vi "subcontrolmotor.vi"(0 "Boolesch":bool) -> ()   [LabVIEW 2011]
uses:
  <vilib>/DAQmx/write.llb/DAQmx Write (Digital Bool 1Line 1Point).vi
  <vilib>/DAQmx/create/channels.llb/DAQmx Create Channel (DO-Digital Output).vi
  <vilib>/DAQmx/miscellaneous.llb/DAQmx Fill In Error Info.vi
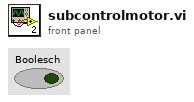
[diagram p1: front panel]
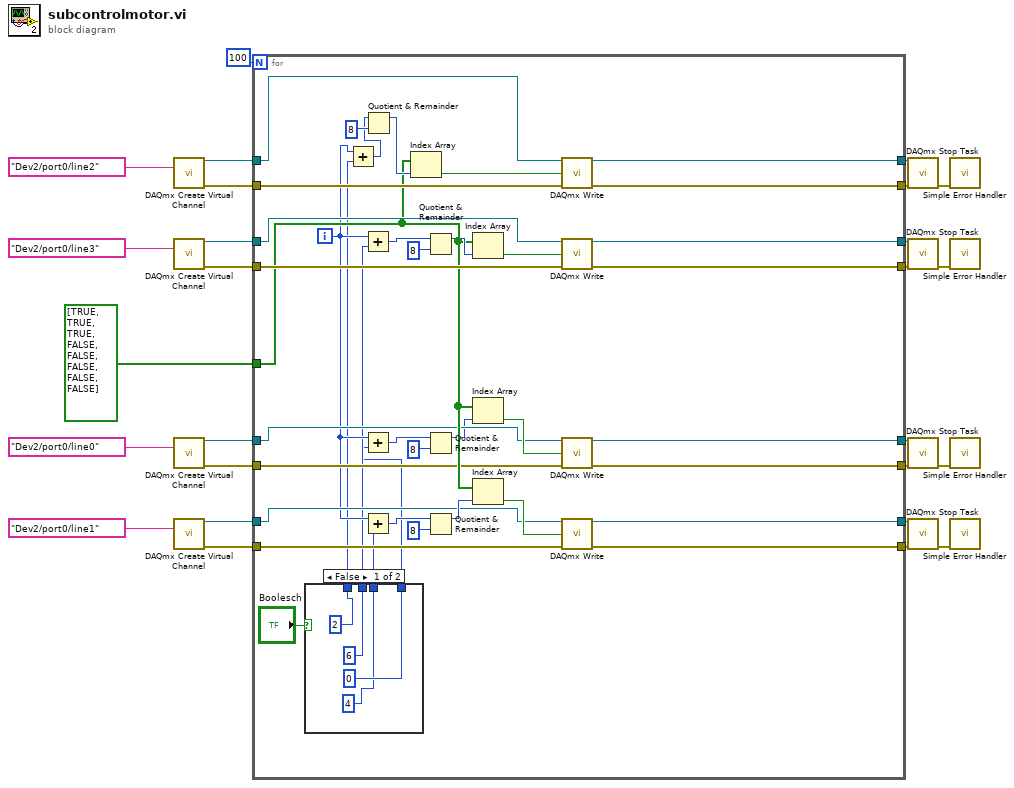
[diagram p0: block diagram]
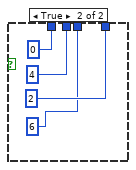
[diagram p2: hidden frame]
diagram:
  n1 = call-poly <vilib>:"DAQmx Create Virtual Channel.vi"("lines"=tag "Dev2/port0/line2") -> ("task out"=w26:refnum<k21>, "error out"=w25:errorcluster)  [unwired: 13 in]
  n2 = call-poly <vilib>:"DAQmx Create Virtual Channel.vi"("lines"=tag "Dev2/port0/line3") -> ("task out"=w20:refnum<k21>, "error out"=w19:errorcluster)  [unwired: 13 in]
  n3 = call-poly <vilib>:"DAQmx Create Virtual Channel.vi"("lines"=tag "Dev2/port0/line0") -> ("task out"=w11:refnum<k21>, "error out"=w10:errorcluster)  [unwired: 13 in]
  n4 = call-poly <vilib>:"DAQmx Create Virtual Channel.vi"("lines"=tag "Dev2/port0/line1") -> ("task out"=w3:refnum<k21>, "error out"=w2:errorcluster)  [unwired: 13 in]
  n5 = for {
    N: 100 -> [_]
    tunnel: w26 -> [w65]
    tunnel: w25 -> [w64]
    tunnel: [w63] -> w24
    tunnel: [w62] -> w22
    tunnel: bool[] [TRUE, TRUE, TRUE, FALSE, FALSE, FALSE, FALSE, FALSE] -> [w50]
    tunnel: w20 -> [w54]
    tunnel: w19 -> [w53]
    tunnel: [w52] -> w17
    tunnel: [w51] -> w16
    tunnel: w11 -> [w47]
    tunnel: w10 -> [w46]
    tunnel: [w45] -> w8
    tunnel: [w44] -> w7
    tunnel: [w43] -> w5
    tunnel: [w42] -> w4
    tunnel: w3 -> [w35]
    tunnel: w2 -> [w34]
    i -> [w33]
    n6 = case shown="False" "Boolesch" {
      tunnel: [2 ("y") 0 ("y")] -> w30
      tunnel: [6 ("y") 4 ("y")] -> w29
      tunnel: [0 ("y") 2 ("y")] -> w28
      tunnel: [4 ("y") 6 ("y")] -> w27
      frame False {
      }
      frame True {
      }
    }
    n7 = Add(x=w33, y=w30) -> (x+y=w32:i32)
    n8 = Add(x=w33, y=w29) -> (x+y=w56:i32)
    n9 = Add(x=w33, y=w28) -> (x+y=w40:i32)
    n10 = Add(x=w33, y=w27) -> (x+y=w41:i32)
    n11 = Quotient & Remainder(x=w32, y=8) -> (x-y*floor(x/y)=w60:i32)  [unwired: 1 out]
    n12 = Index Array(array=w50, index=w60) -> (element=w59:bool)
    n13 = Quotient & Remainder(x=w56, y=8) -> (x-y*floor(x/y)=w58:i32)  [unwired: 1 out]
    n14 = Quotient & Remainder(x=w40, y=8) -> (x-y*floor(x/y)=w38:i32)  [unwired: 1 out]
    n15 = Quotient & Remainder(x=w41, y=8) -> (x-y*floor(x/y)=w39:i32)  [unwired: 1 out]
    n16 = Index Array(array=w50, index=w58) -> (element=w55:bool)
    n17 = Index Array(array=w50, index=w38) -> (element=w48:bool)
    n18 = Index Array(array=w50, index=w39) -> (element=w49:bool)
    n19 = call-poly <vilib>:"DAQmx Write.vi"("task/channels in"=w65, "data"=w59, "error in"=w64) -> ("task out"=w62:refnum<k21>, "error out"=w63:errorcluster)  [unwired: 10 in, 1 out]
    n20 = call-poly <vilib>:"DAQmx Write.vi"("task/channels in"=w54, "data"=w55, "error in"=w53) -> ("task out"=w52:refnum<k21>, "error out"=w51:errorcluster)  [unwired: 10 in, 1 out]
    n21 = call-poly <vilib>:"DAQmx Write.vi"("task/channels in"=w47, "data"=w48, "error in"=w46) -> ("task out"=w45:refnum<k21>, "error out"=w44:errorcluster)  [unwired: 10 in, 1 out]
    n22 = call-poly <vilib>:"DAQmx Write.vi"("task/channels in"=w35, "data"=w49, "error in"=w34) -> ("task out"=w43:refnum<k21>, "error out"=w42:errorcluster)  [unwired: 10 in, 1 out]
  }
  n23 = call <vilib>:"DAQmx Stop Task.vi"("task/channels in"=w22, "error in"=w24) -> ("error out"=w23:errorcluster)  [unwired: 12 in, 1 out]
  n24 = call <vilib>:"DAQmx Stop Task.vi"("task/channels in"=w17, "error in"=w16) -> ("error out"=w18:errorcluster)  [unwired: 12 in, 1 out]
  n25 = call <vilib>:"DAQmx Stop Task.vi"("task/channels in"=w8, "error in"=w7) -> ("error out"=w9:errorcluster)  [unwired: 12 in, 1 out]
  n26 = call <vilib>:"DAQmx Stop Task.vi"("task/channels in"=w5, "error in"=w4) -> ("error out"=w6:errorcluster)  [unwired: 12 in, 1 out]
  n27 = call <vilib>:"Simple Error Handler.vi"("error in (no error)"=w23) -> ()  [unwired: 4 in, 5 out]
  n28 = call <vilib>:"Simple Error Handler.vi"("error in (no error)"=w18) -> ()  [unwired: 4 in, 5 out]
  n29 = call <vilib>:"Simple Error Handler.vi"("error in (no error)"=w9) -> ()  [unwired: 4 in, 5 out]
  n30 = call <vilib>:"Simple Error Handler.vi"("error in (no error)"=w6) -> ()  [unwired: 4 in, 5 out]
